vi "Configuration Current.vi"(0 "VISA resource name":refnum<visa-resource-name>, 1 "Channel 1-8 (0:Ch1)":u8(ring) items=["Channel 1", "Channel 2", "Channel 3", "Channel 4", "Channel 5", "Channel 6", "Channel 7", "Channel 8 "], 3 "Level 1 (5.0)":sgl=5.0 min=0 format="%.4f", 4 "Level 2 (0.0)":sgl min=0 format="%.4f", 5 "error in (no error)":errorcluster, 6 "High/Low (1:High)":u8(slide)=1 scale=0.0..1.0, 7 "Static/Dynamic (0:Static)":u8(slide) scale=0.0..1.0, 8 "Voltage Range(V) (16.0)":sgl=16.0 min=0 format="%.2f", 10 "Rise (3.2)":sgl=3.2 min=0 step=0.32 format="%.2f", 11 "T1 (0.0)":sgl format="%.2f", 12 "Fall (3.2)":sgl=3.2 min=0 step=0.32 format="%.2f", 13 "T2 (0.0)":sgl format="%.2f") -> (14 "VISA resource name out":refnum<visa-resource-name>, 19 "error out":errorcluster)   [LabVIEW 2015, in "Chroma ATE 6310.lvlib"]
doc: "This function sets the constant current mode.\n\nIn CC mode, the Load will sink a current in accordance with the programmed value regardless of input voltage."
uses:
  <instrlib>/Chroma ATE 6310/Chroma ATE 6310.lvlib
panel:
  # "Duration \nParameter(mS)"
  # "Current Level(A)"
  # "Slew Rate\n(mA/uS)"
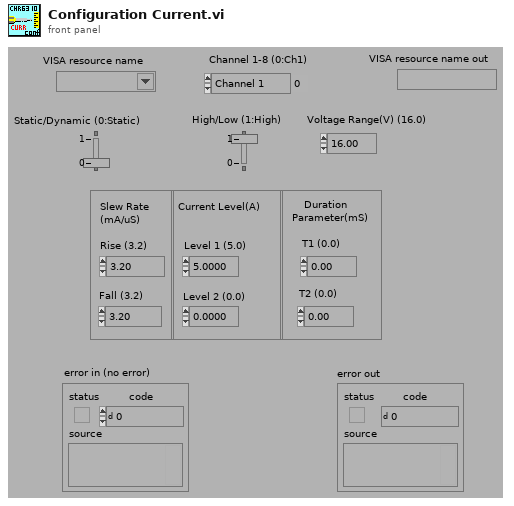
[diagram p1: front panel]
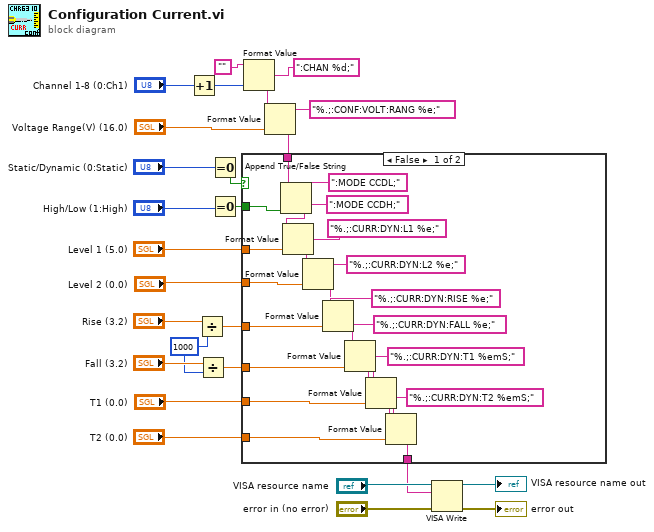
[diagram p0: block diagram]
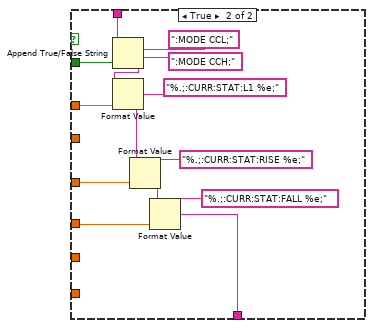
[diagram p2: hidden frame]
diagram:
  w12 = 1000
  n1 = Increment(x="Channel 1-8 (0:Ch1)") -> (x+1=w20:u8)
  n2 = Divide(x="Rise (3.2)", y=w12) -> (x/y=w15:sgl)
  n3 = Divide(x="Fall (3.2)", y=w12) -> (x/y=w13:sgl)
  n4 = Equal To 0?(x="Static/Dynamic (0:Static)") -> (x = 0?=w23:bool)
  n5 = Equal To 0?(x="High/Low (1:High)") -> (x = 0?=w17:bool)
  n6 = Format Value(string ("")="", format string=":CHAN %d;", value (0)=w20) -> (output string=w3:string)
  n7 = Format Value(string ("")=w3, format string="%.;:CONF:VOLT:RANG %e;", value (0)="Voltage Range(V) (16.0)") -> (output string=w1:string)
  n8 = case shown="False" w23 {
    tunnel: w1 -> [w34 w55]
    tunnel: "Level 1 (5.0)" -> [w44 w57]
    tunnel: [w39 w59] -> w5
    tunnel: "Level 2 (0.0)" -> [w38 _]
    tunnel: w17 -> [w35 w56]
    tunnel: w15 -> [w31 w51]
    tunnel: w13 -> [w30 w50]
    tunnel: "T1 (0.0)" -> [w29 _]
    tunnel: "T2 (0.0)" -> [w28 _]
    frame False {
      n9 = Append True/False String(1:w35, 2:":MODE CCDH;", 3:":MODE CCDL;", 4:w34) -> (0:w32:string)
      n10 = Format Value(string ("")=w32, format string="%.;:CURR:DYN:L1 %e;", value (0)=w44) -> (output string=w49:string)
      n11 = Format Value(string ("")=w49, format string="%.;:CURR:DYN:L2 %e;", value (0)=w38) -> (output string=w43:string)
      n12 = Format Value(string ("")=w43, format string="%.;:CURR:DYN:RISE %e;", value (0)=w31) -> (output string=w47:string)
      n13 = Format Value(string ("")=w47, format string="%.;:CURR:DYN:FALL %e;", value (0)=w30) -> (output string=w42:string)
      n14 = Format Value(string ("")=w42, format string="%.;:CURR:DYN:T1 %emS;", value (0)=w29) -> (output string=w41:string)
      n15 = Format Value(string ("")=w41, format string="%.;:CURR:DYN:T2 %emS;", value (0)=w28) -> (output string=w39:string)
    }
    frame True {
      n16 = Append True/False String(1:w56, 2:":MODE CCH;", 3:":MODE CCL;", 4:w55) -> (0:w52:string)
      n17 = Format Value(string ("")=w52, format string="%.;:CURR:STAT:L1 %e;", value (0)=w57) -> (output string=w58:string)
      n18 = Format Value(string ("")=w58, format string="%.;:CURR:STAT:RISE %e;", value (0)=w51) -> (output string=w62:string)
      n19 = Format Value(string ("")=w62, format string="%.;:CURR:STAT:FALL %e;", value (0)=w50) -> (output string=w59:string)
    }
  }
  n20 = VISA Write(VISA resource name="VISA resource name", write buffer=w5, error in (no error)="error in (no error)") -> (VISA resource name out=→"VISA resource name out":refnum<visa-resource-name>, error out=→"error out":errorcluster)  [unwired: 1 out]
